vi "Obtain SPI CS.vi"(5 "Purpose (\"SPI CS\")":string="SPI CS", 7 "CS GPIO":T1=5, 8 "error in (no error)":errorcluster, 10 "CS Active Low (T)":bool=TRUE, 11 "Session in":refnum<class "Session.lvclass">) -> (0 "error out":errorcluster, 3 "Session out":refnum<class "Session.lvclass">)   [LabVIEW 2020, in "CTI.lvlib" / "Session.lvclass"]
uses:
  Session.lvclass
  Session.lvclass/Session.ctl
  GPIO Direction.ctl
  CTI.lvlib
  SPI CS/SPI CS.lvclass
  9e492bde-7e1e-4053-b97c-863c07586c82.vi
  GPIO Number.ctl
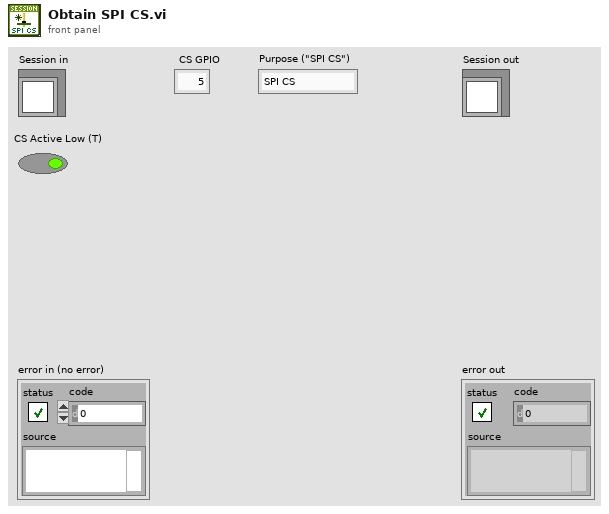
[diagram p1: front panel]
types:
  T1 = typedef "CTI.lvlib/GPIO Number.ctl" = i8
  T2 = typedef "CTI.lvlib/GPIO Direction.ctl" = enum16{"In", "Out"}
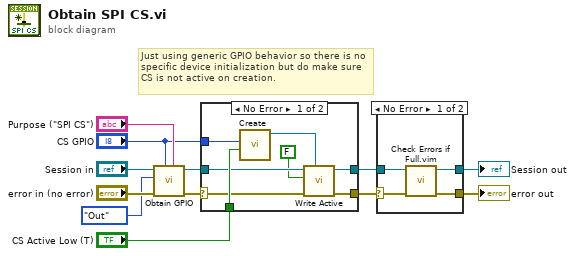
[diagram p0: block diagram]
diagram:
  # "Just using generic GPIO behavior so there is no specific device initialization but do make sure CS is not active on creation."
  n1 = call "Obtain GPIO.vi"("Purpose (\"GPIO\")"="Purpose (\"SPI CS\")", "GPIO #"="CS GPIO", "error in (no error)"="error in (no error)", "GPIO Direction"=GPIO_Direction."Out", "Session in"="Session in") -> ("error out"=w8:errorcluster, "Session out"=w7:refnum<class "Session.lvclass">)  [unwired: 5 in]
  n2 = case shown="No Error" w8 {
    selector: w8 -> [w17 w21]
    tunnel: w7 -> [w18 w22]
    tunnel: "CS Active Low (T)" -> [w20 _]
    tunnel: [w15 w22] -> w5
    tunnel: [w14 w21] -> w4
    tunnel: "CS GPIO" -> [w13 _]
    frame No Error {
      n3 = call "Create.vi"("CS Active Low"=w20, "GPIO"=w13) -> ("SPI CS out"=w19:refnum<class "SPI CS.lvclass">)  [unwired: 8 in, 1 out]
      n4 = call "Write Active.vi"("SPI CS"=w19, "error in (no error)"=w17, "Active"=FALSE, "Session In"=w18) -> ("error out"=w14:errorcluster, "Session Out"=w15:refnum<class "Session.lvclass">)  [unwired: 6 in]
    }
    frame Error {
    }
  }
  n5 = case shown="No Error" w4 {
    selector: w4 -> [w25 w27]
    tunnel: w5 -> [w26 w28]
    tunnel: [w24 w28] -> w3
    tunnel: [w23 w27] -> w2
    frame No Error {
      n6 = call "Check Errors if Full.vim"("error in (no error)"=w25, "Session in"=w26) -> ("error out"=w23:errorcluster, "Session out"=w24:refnum<class "Session.lvclass">)  [unwired: 8 in]
    }
    frame Error {
    }
  }
  "error out" <- w2
  "Session out" <- w3
